vi "ReadWriteTest.vi"() -> ()   [LabVIEW 2013]
panel:
  out "return count":u32
  out "Bytes":u32
  in  "write buffer":string
  out "read buffer":string
  in  "stop":bool
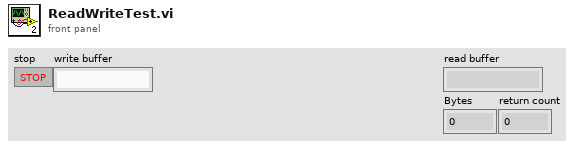
[diagram p1: front panel]
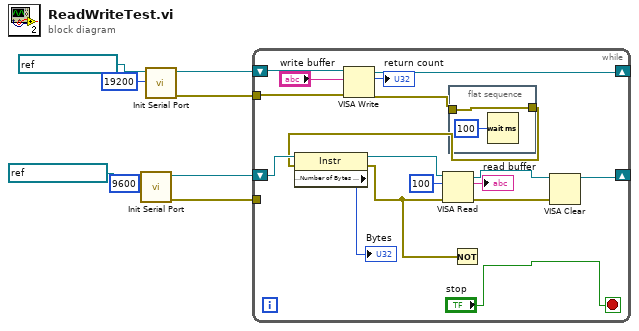
[diagram p0: block diagram]
diagram:
  n1 = call "Init Serial Port.vi"("baud rate"=u32 9600, "VISA Refnum in"=refnum<visa-resource-name> "ASRL1::INSTR") -> ("error out"=w2:errorcluster, "VISA Refnum out"=w3:refnum<visa-resource-name>)  [unwired: 8 in]
  n2 = call "Init Serial Port.vi"("baud rate"=u32 19200, "VISA Refnum in"=refnum<visa-resource-name> "ASRL2::INSTR") -> ("error out"=w1:errorcluster, "VISA Refnum out"=w4:refnum<visa-resource-name>)  [unwired: 8 in]
  n3 = while {
    tunnel: w2 -> [_]
    tunnel: w1 -> [w24]
    shift-right: [w18] -> _
    shift-left: w3 -> [w17]
    shift-right: [w14] -> _
    shift-left: w4 -> [w25]
    stop <- "stop" stop-if-true
    n4 = property class="Instr"(reference=w17, error in=w12) -> (reference out=w16:refnum<visa-resource-name>, error out=w10:errorcluster, "Serial Settings:Number of Bytes at Serial Port"=→"Bytes":u32)
    n5 = VISA Write(VISA resource name=w25, write buffer="write buffer", error in (no error)=w24) -> (VISA resource name out=w14:refnum<visa-resource-name>, return count=→"return count":u32, error out=w13:errorcluster)
    n6 = VISA Read(VISA resource name=w16, byte count=u32 100, error in (no error)=w10) -> (VISA resource name out=w20:refnum<visa-resource-name>, read buffer=→"read buffer":string, error out=w19:errorcluster)  [unwired: 1 out]
    n7 = flat-sequence {
      tunnel: w13 -> [w27]
      tunnel: [w27] -> w12
      frame #0 {
        n8 = Wait (ms)(milliseconds to wait=u32 100) -> ()  [unwired: 1 out]
      }
    }
    n9 = Not(x=w10) -> ()  [unwired: 1 out]
    n10 = VISA Clear(VISA resource name=w20, error in (no error)=w19) -> (VISA resource name out=w18:refnum<visa-resource-name>)  [unwired: 1 out]
  }
